vi "动态更新表格.vi"(5 "行数":i32, 7 "Tbl引用句柄":refnum<vi>, 8 "error in (no error)":errorcluster caption="错误输入（无错误）", 10 "当前数值":string[](array[string]), 11 "枚举":enum16{"初始化", "更新"}(ring)=enum."更新") -> (0 "error out":errorcluster caption="错误输出")   [LabVIEW 2014, in "表格.lvlib"]
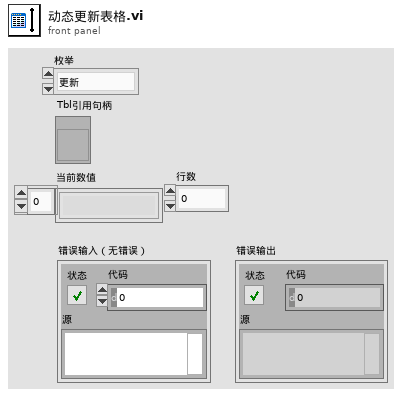
[diagram p1: front panel]
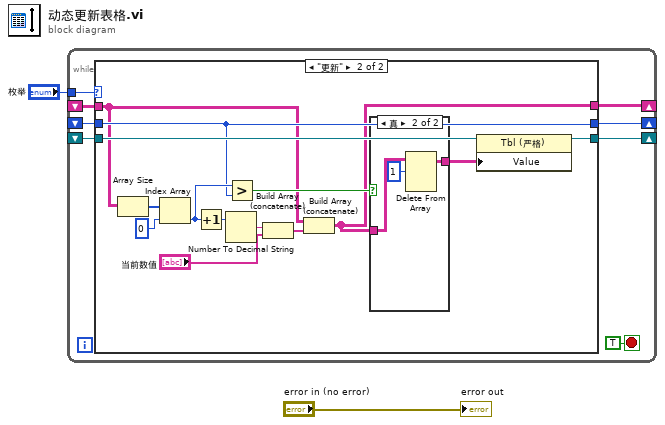
[diagram p0: block diagram]
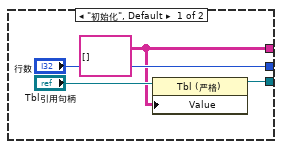
[diagram p2: hidden frame]
diagram:
  n1 = while {
    tunnel: "枚举" -> [w9]
    shift-right: [w8] -> _
    shift-left: _ -> [w4]
    shift-right: [w7] -> _
    shift-left: _ -> [w3]
    shift-right: [w6] -> _
    shift-left: _ -> [w5]
    stop <- TRUE stop-if-true
    n2 = case shown="\"更新\"" w9 {
      tunnel: [w11 w15] -> w8
      tunnel: ["行数" w18] -> w7
      tunnel: [w13 w27] -> w6
      tunnel: w5 -> [_ w28]
      tunnel: w4 -> [_ w17]
      tunnel: w3 -> [_ w18]
      frame "初始化", Default {
        w11 = string[][] []
        n3 = property class="Tbl (严格)"(reference="Tbl引用句柄", "Value"=w11) -> (reference out=w13:refnum<vi>)  [unwired: 1 in, 1 out]
      }
      frame "更新" {
        n4 = Array Size(array=w17) -> (size(s)=w26:i32[])
        n5 = Index Array(array=w26, index=0 ("索引")) -> (element=w21:i32)
        n6 = Increment(x=w21) -> (x+1=w24:i32)
        n7 = Number To Decimal String(number=w24) -> (decimal integer string=w23:string)  [unwired: 1 in]
        n8 = Greater?(x=w21, y=w18) -> (0:w20:bool)
        n9 = Build Array (concatenate)(w23, "当前数值") -> (w19:string[])
        n10 = Build Array (concatenate)(w17, w19) -> (w15:string[][])
        n11 = case shown="真" w20 {
          tunnel: w15 -> [w29 w32]
          tunnel: [w29 w30] -> w16
          frame False {
          }
          frame True {
            n12 = Delete From Array(array=w32, length=1 ("长度")) -> (array with subset deleted=w30:string[][])  [unwired: 2 in, 1 out]
          }
        }
        n13 = property class="Tbl (严格)"(reference=w28, "Value"=w16) -> (reference out=w27:refnum<vi>)  [unwired: 1 in, 1 out]
      }
    }
  }
  "error out" <- "error in (no error)"
